vi "Roc_Auc_Score.vi"(8 "error in (no error)":errorcluster caption="entrée d'erreur (pas d'erreur)", 9 "y_score":string[][](array[string]), 10 "y_true":string[][](array[string]), 11 "roc_auc_score":T1={"average"="macro", "sample_weight"=[], "max_fpr"="None", "multi_class"="raise", "labels"=["None"]}) -> (0 "error out":errorcluster caption="sortie d'erreur", 3 "Score":string)   [LabVIEW 2020]
doc: "Compute Area Under the Receiver Operating Characteristic Curve (ROC AUC) from prediction scores.\n\nNote : this implementation can be used with binary, multiclass and multilabel classification, but some restrictions apply (see Parameters).\n\n\n\nParameters : \n\n- y_true : array-like of shape (n_samples,) or (n_samples, n_classes)\nTrue labels or binary label indicators. The binary and multiclass cases expect labels with shape (n_samples,) while the multilabel case expects binary label indicators with shape (n_samples, n_classes).\n\n- y_score : array-like of shape (n_samples,) or (n_samples, n_classes)\nTarget scores. In the binary and multilabel cases, these can be either probability estimates or non-thresholded decision values (as returned by decision_function on some classifiers). In the multiclass case, these must be probability estimates which sum to 1. The binary case expects a shape (n_samples,), and the scores must be the scores of the class with the greater label. The multiclass and multilabel cases expect a shape (n_samples, n_classes). In the multiclass case, the order of the class scores must correspond to the order of labels, if provided, or else to the numerical or lexicographical order of the labels in y_true.\n\n- average : {‘micro’, ‘macro’, ‘samples’, ‘weighted’} or None, default=’macro’\nIf None, the scores for each class are returned. Otherwise, this determines the type of averaging performed on the data: Note: multiclass ROC AUC currently only handles the ‘macro’ and ‘weighted’ averages.\n\n'micro':\nCalculate metrics globally by considering each element of the label indicator matrix as a label.\n\n'macro':\nCalculate metrics for each label, and find their unweighted mean. This does not take label imbalance into account.\n\n'weighted':\nCalculate metrics for each label, and find their average, weighted by support (the number of true instances for each label).\n\n'samples':\nCalculate metrics for each instance, and find their average.\n\nWill be ignored when y_true is binary.\n\n- sample_weight : array-like of shape (n_samples,), default=None\nSample weights.\n\n- max_fpr : float > 0 and <= 1, default=None\nIf not None, the standardized partial AUC [2] over the range [0, max_fpr] is returned. For the multiclass case, max_fpr, should be either equal to None or 1.0 as AUC ROC partial computation currently is not supported for multiclass.\n\n- multi_class : {‘raise’, ‘ovr’, ‘ovo’}, default=’raise’\nMulticlass only. Determines the type of configuration to use. The default value raises an error, so either 'ovr' or 'ovo' must be passed explicitly.\n\n'ovr':\nComputes the AUC of each class against the rest [3] [4]. This treats the multiclass case in the same way as the multilabel case. Sensitive to class imbalance even when average == 'macro', because class imbalance affects the composition of each of the ‘rest’ groupings.\n\n'ovo':\nComputes the average AUC of all possible pairwise combinations of classes [5]. Insensitive to class imbalance when average == 'macro'.\n\n- labels : array-like of shape (n_classes,), default=None\nMulticlass only. List of labels that index the classes in y_score. If None, the numerical or lexicographical order of the labels in y_true is used.\n\n\nReturns : \n\n- auc : float"
uses:
  Roc_Auc_Score.lvclass
panel:
  out "Roc_Auc_Score.lvclass":refnum<class "Roc_Auc_Score.lvclass">
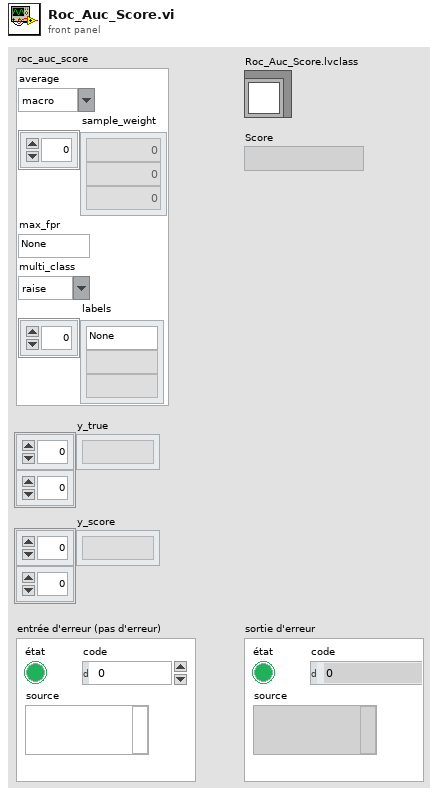
[diagram p1: front panel]
types:
  T1 = cluster{"average":string, "sample_weight":dbl[], "max_fpr":string, "multi_class":string, "labels":string[]}
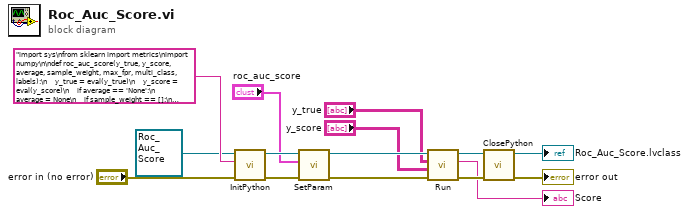
[diagram p0: block diagram]
diagram:
  n1 = call-dynamic "InitPython.vi"("error in (no error)"="error in (no error)", "Python Instruction"="import sys\nfrom sklearn import metrics\nimport numpy\n\ndef roc_auc_score(y_true, y_score, average, sample_weight, max_fpr, multi_class, labels):\n    y_true = eval(y_true)\n    y_score = eval(y_score)\n    if average == 'None':\n        average = None\n    if sample_weight == []:\n        sample_weight = None\n    if max_fpr == 'None':\n        max_fpr = None\n    else:\n        max_fpr = eval(max_fpr)\n    if labels == [] or labels[0] == 'None':\n        labels = None\n    try:\n        roc_auc_score = metrics.roc_auc_score(y_true, y_score, average, sample_weight, max_fpr, multi_class, labels)\n        roc_auc_score = roc_auc_score.tolist()\n        return str(roc_auc_score)\n    except:\n        erreur = sys.exc_info()\n        typerr = u\"%s\" % (erreur[0])\n        typerr = typerr[typerr.find(\"'\")+1:typerr.rfind(\"'\")]\n        msgerr = u\"%s\" % (erreur[1])\n        message = str('/!\\\\ {0} : {1}'. format(typerr,msgerr))\n        return message", "Scikit-learn en entrée"=refnum<class "Roc_Auc_Score.lvclass"> refnum ("Roc_Auc_Score.lvclass")) -> ("error out"=w11:errorcluster, "Scikit-learn en sortie"=w10:refnum<class "Roc_Auc_Score.lvclass">)  [unwired: 7 in]
  n2 = call-dynamic "SetParam.vi"("error in (no error)"=w11, "roc_auc_score"="roc_auc_score", "Roc_Auc_Score.lvclass"=w10) -> ("error out"=w7:errorcluster, "Roc_Auc_Score.lvclass"=w8:refnum<class "Roc_Auc_Score.lvclass">)  [unwired: 7 in]
  n3 = call-dynamic "Run.vi"("error in (no error)"=w7, "y_score"="y_score", "y_true"="y_true", "Roc_Auc_Score.lvclass"=w8) -> ("error out"=w6:errorcluster, "String Data"=→"Score":string, "Roc_Auc_Score.lvclass"=w5:refnum<class "Roc_Auc_Score.lvclass">)  [unwired: 5 in]
  n4 = call-dynamic "ClosePython.vi"("error in (no error)"=w6, "Scikit-learn en entrée"=w5) -> ("error out"=→"error out":errorcluster, "Scikit-learn en sortie"=→"Roc_Auc_Score.lvclass":refnum<class "Roc_Auc_Score.lvclass">)  [unwired: 8 in]
